vi "Initialize VeriStand Globals_stub.vi"(8 "error in (no error)":errorcluster) -> (0 "error out":errorcluster)   [LabVIEW 2019]
uses:
  <vilib>/NI VeriStand/Custom Device API/Data Table Ref.ctl
  <vilib>/NI VeriStand/Custom Device API/Global Data Refs.vi
  <vilib>/NI VeriStand/Custom Device API/Custom Device API.lvlib
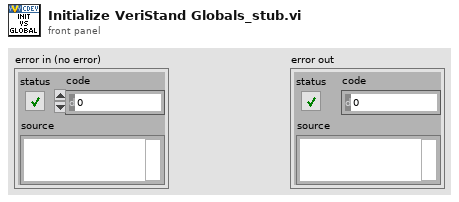
[diagram p1: front panel]
types:
  T1 = typedef "Custom Device API.lvlib/Data Table Ref.ctl" = cluster{"Ptr.Beg":u64, "Ptr.End":u64}
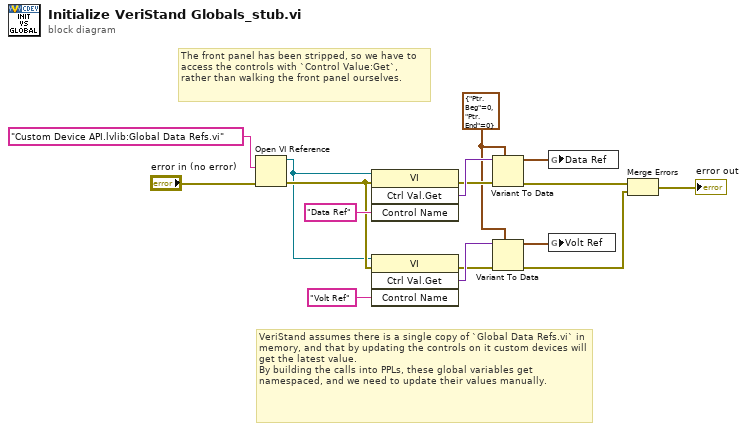
[diagram p0: block diagram]
diagram:
  w3 = T1 {"Ptr.Beg"=0, "Ptr.End"=0} ("Data Table Ref")
  # "The front panel has been stripped, so we have to access the controls with `Control Value:Get`, rather than walking the front panel ourselves."
  # "VeriStand assumes there is a single copy of `Global Data Refs.vi` in memory, and that by updating the controls on it custom devices will get the latest value. \nBy building the calls into PPLs, these global variables get namespaced, and we need to update their values manually."
  n1 = Open VI Reference(vi path="Custom Device API.lvlib:Global Data Refs.vi", error in (no error)="error in (no error)") -> (vi reference=w6:refnum<vi>, error out=w8:errorcluster)  [unwired: 4 in]
  n2 = invoke class="VI" method="Ctrl Val.Get"(reference=w6, error in=w8, "Control Name"="Data Ref" ("y")) -> (error out=w9:errorcluster, "Get Control Value Variant"=w10:variant)  [unwired: 1 in, 2 out]
  n3 = invoke class="VI" method="Ctrl Val.Get"(reference=w6, error in=w8, "Control Name"="Volt Ref" ("y")) -> (error out=w4:errorcluster, "Get Control Value Variant"=w5:variant)  [unwired: 1 in, 2 out]
  n4 = Variant To Data(error in=w9, type=w3, Variant=w10) -> (data=w1:T1, error out=w13:errorcluster)
  n5 = Variant To Data(error in=w4, type=w3, Variant=w5) -> (data=w2:T1, error out=w12:errorcluster)
  n6 = global write "Global Data Refs.vi" "Data Ref"(w1) -> ()
  n7 = global write "Global Data Refs.vi" "Volt Ref"(w2) -> ()
  n8 = Merge Errors(w13, w12) -> (→"error out":errorcluster)
